vi "ScreenShot.vi"() -> ()   [LabVIEW 2016]
panel:
  in  "vi path":path
  in  "error in (no error)":errorcluster
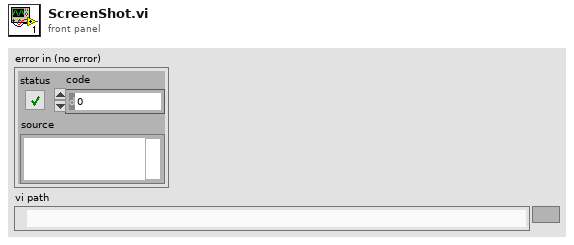
[diagram p1: front panel]
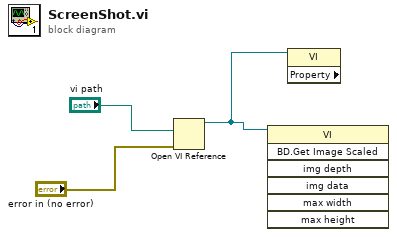
[diagram p0: block diagram]
diagram:
  n1 = Open VI Reference(vi path="vi path", error in (no error)="error in (no error)") -> (vi reference=w1:refnum<vi>)  [unwired: 4 in, 1 out]
  n2 = invoke class="VI" method="BD.Get Image Scaled"(reference=w1) -> ()  [unwired: 6 in, 7 out]
  n3 = property class="VI" props=[](reference=w1) -> ()  [unwired: 1 in, 3 out]
